vi "SystemToggleLevitationControl (1).vi"(11 "LevitationControl":bool) -> ()   [LabVIEW 2017]
doc: "Writes to all solenoids associated with Levitation."
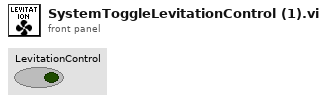
[diagram p1: front panel]
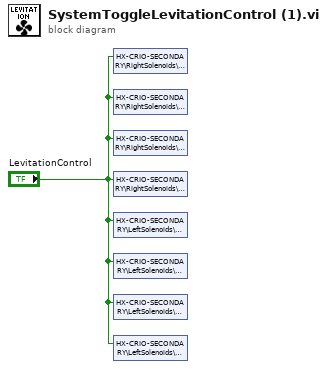
[diagram p0: block diagram]
diagram:
  n1 = shared-variable "HX-CRIO-SECONDARY\\RightSolenoids\\NC08"("LevitationControl") -> ()  [unwired: 1 in, 1 out]
  n2 = shared-variable "HX-CRIO-SECONDARY\\RightSolenoids\\NC05"("LevitationControl") -> ()  [unwired: 1 in, 1 out]
  n3 = shared-variable "HX-CRIO-SECONDARY\\RightSolenoids\\NC06"("LevitationControl") -> ()  [unwired: 1 in, 1 out]
  n4 = shared-variable "HX-CRIO-SECONDARY\\RightSolenoids\\NC07"("LevitationControl") -> ()  [unwired: 1 in, 1 out]
  n5 = shared-variable "HX-CRIO-SECONDARY\\LeftSolenoids\\NC03"("LevitationControl") -> ()  [unwired: 1 in, 1 out]
  n6 = shared-variable "HX-CRIO-SECONDARY\\LeftSolenoids\\NC04"("LevitationControl") -> ()  [unwired: 1 in, 1 out]
  n7 = shared-variable "HX-CRIO-SECONDARY\\LeftSolenoids\\NC02"("LevitationControl") -> ()  [unwired: 1 in, 1 out]
  n8 = shared-variable "HX-CRIO-SECONDARY\\LeftSolenoids\\NC01"("LevitationControl") -> ()  [unwired: 1 in, 1 out]
